vi "MyG#G3Templ_GetAttributes.vi"(0 "reference in":refnum<class "MyG#G3Templ.lvclass">, 1 "return data":bool=TRUE, 5 "error in (no error)":errorcluster) -> (14 "reference out":refnum<class "MyG#G3Templ.lvclass">, 15 "attributes ref":T2, 16 "attributes":T1, 19 "error out":errorcluster)   [LabVIEW 2020, in "MyG#G3Templ.lvclass"]
doc: "Returns a reference and if wanted the actual data values of the attributes. This method is used by the subclasses to access parent attributes."
uses:
  MyG#G3Templ.lvclass
  ObjectAttributesRef.ctl
  protected/ObjectAttributes.ctl
  MyG#G3Templ.lvclass/MyG#G3Templ.ctl
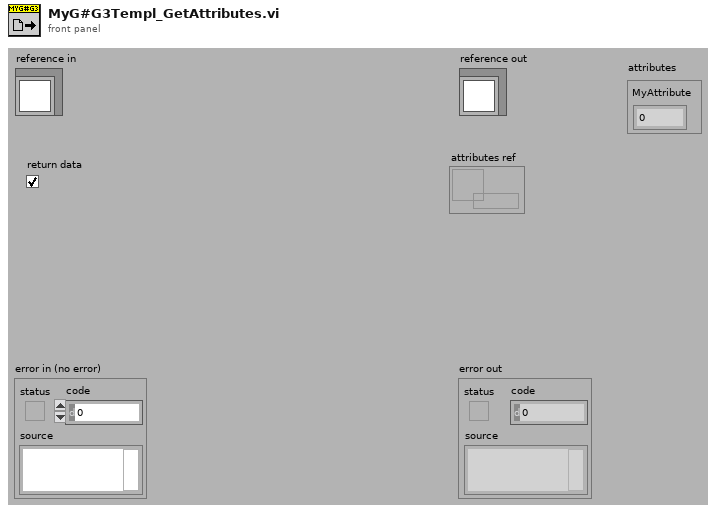
[diagram p1: front panel]
types:
  T1 = typedef "MyG#G3Templ.lvclass/ObjectAttributes.ctl" = cluster{"MyAttribute":dbl}
  T2 = typedef "MyG#G3Templ.lvclass/ObjectAttributesRef.ctl" = refnum<data-value>
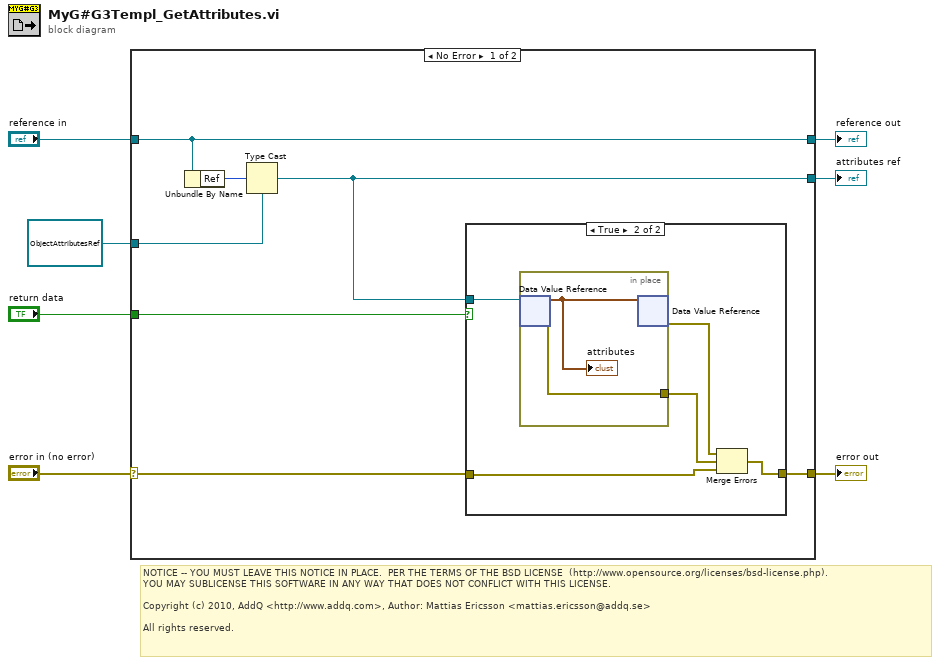
[diagram p0: block diagram]
diagram:
  # "NOTICE -- YOU MUST LEAVE THIS NOTICE IN PLACE.  PER THE TERMS OF THE BSD LICENSE  (http://www.opensource.org/licenses/bsd-license.php).\nYOU MAY SUBLICENSE THIS SOFTWARE IN ANY WAY THAT DOES NOT CONFLICT WITH THIS LICENSE.\n\nCopyright (c) 2010, AddQ <http://www.addq.com>, Author: Mattias Ericsson <mattias.ericsson@addq.se>\n\nAll rights reserved."
  n1 = case shown="No Error" "error in (no error)" {
    selector: "error in (no error)" -> [w12 w25]
    tunnel: [w11 w25] -> w6
    tunnel: [w14 w24] -> w4
    tunnel: "reference in" -> [w14 w24]
    tunnel: [w10 w23] -> w3
    tunnel: "return data" -> [w13 _]
    tunnel: T2 refnum ("attributes ref") -> [w8 w23]
    frame No Error {
      n2 = Unbundle By Name(w14) -> ("Ref"=w9:u32)
      n3 = Type Cast(type=w8, x=w9) -> (*(type *) &x=w10:T2)
      n4 = case shown="True" w13 {
        tunnel: w10 -> [_ w20]
        tunnel: w12 -> [w15 w19]
        tunnel: [w15 w16] -> w11
        frame False {
        }
        frame True {
          n5 = in-place {
            in-place-border: [w22] -> w18
            n6 = in-place-dvr #1(w20) -> (w21:T1, w22:errorcluster)
            "attributes" <- w21
            n7 = in-place-dvr #1(w21) -> (w17:errorcluster)  [unwired: 1 out]
          }
          n8 = Merge Errors(w17, w18, w19) -> (w16:errorcluster)
        }
      }
    }
    frame Error {
    }
  }
  "error out" <- w6
  "reference out" <- w4
  "attributes ref" <- w3
